vi "Exit.vi"(8 "error in (no error)":errorcluster, 11 "Active in":refnum<class "Active.lvclass">) -> (0 "error out":errorcluster, 3 "Active out":refnum<class "Active.lvclass">)   [LabVIEW 2024, in "Active.lvlib" / "Active.lvclass"]
uses:
  Active.lvclass
  Active.lvclass/Active.ctl
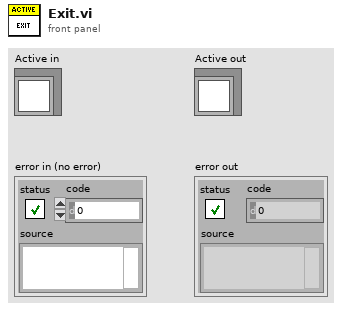
[diagram p1: front panel]
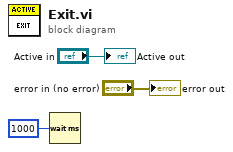
[diagram p0: block diagram]
diagram:
  n1 = Wait (ms)(milliseconds to wait=u32 1000) -> ()  [unwired: 1 out]
  "error out" <- "error in (no error)"
  "Active out" <- "Active in"
